vi "Test CAN read.vi"() -> ()   [LabVIEW 2023, in "PCAN API.lvlib"]
uses:
  PCAN API.lvlib
panel:
  out "MessageBuffer out 2":T1
  out "error out 3":errorcluster
  out "Array":errorcluster[](array[cluster])
  out "error out 2":errorcluster
  out "error out":errorcluster
  out "MessageBuffer out":T2(array[cluster])
  in  "stop":bool
  in  "error in":errorcluster
  in  "Channel":u16=81 format="%x"
  in  "IOPort":u32 format="%x"
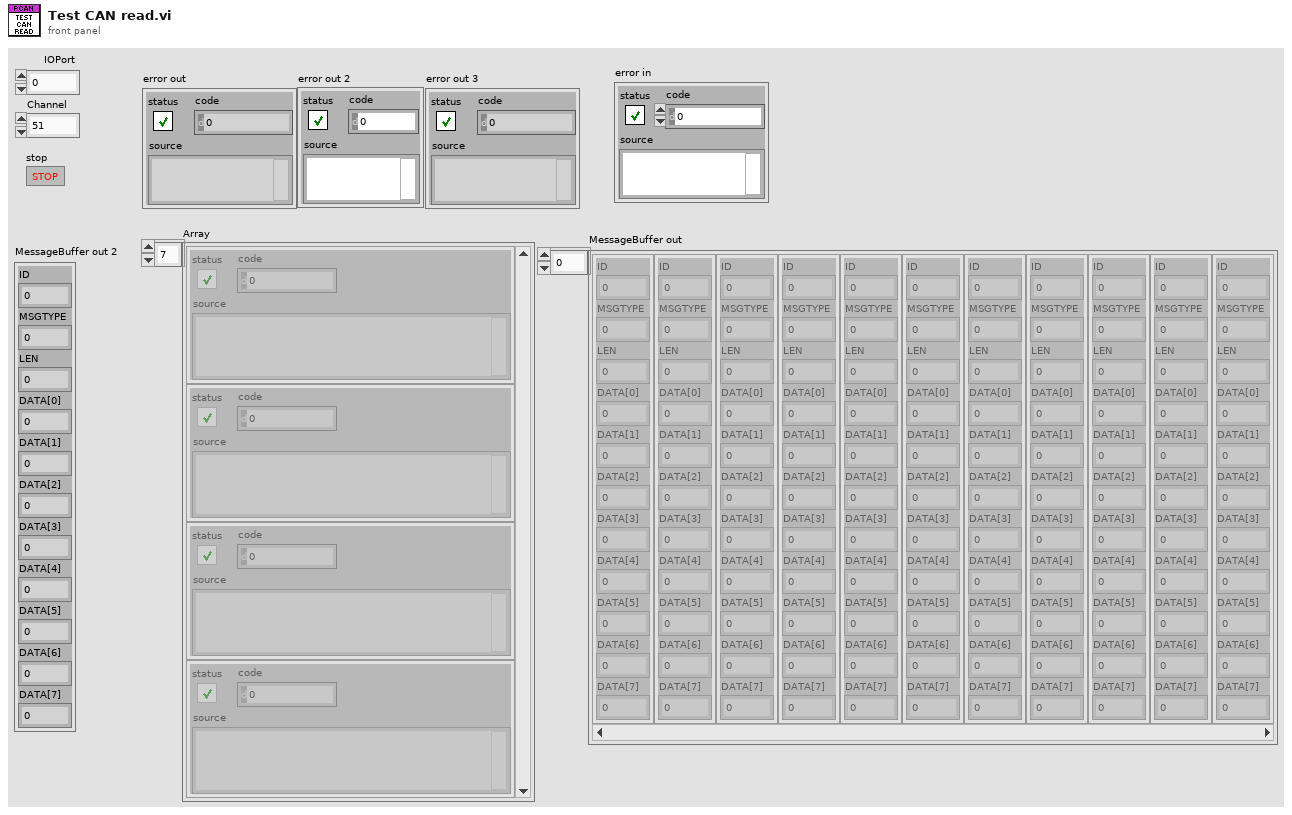
[diagram p1: front panel]
types:
  T1 = cluster{"ID":u32, "MSGTYPE":u8, "LEN":u8, "DATA[0]":u8, "DATA[1]":u8, "DATA[2]":u8, "DATA[3]":u8, "DATA[4]":u8, "DATA[5]":u8, "DATA[6]":u8, "DATA[7]":u8}
  T2 = cluster{"ID":u32, "MSGTYPE":u8, "LEN":u8, "DATA[0]":u8, "DATA[1]":u8, "DATA[2]":u8, "DATA[3]":u8, "DATA[4]":u8, "DATA[5]":u8, "DATA[6]":u8, "DATA[7]":u8}[]
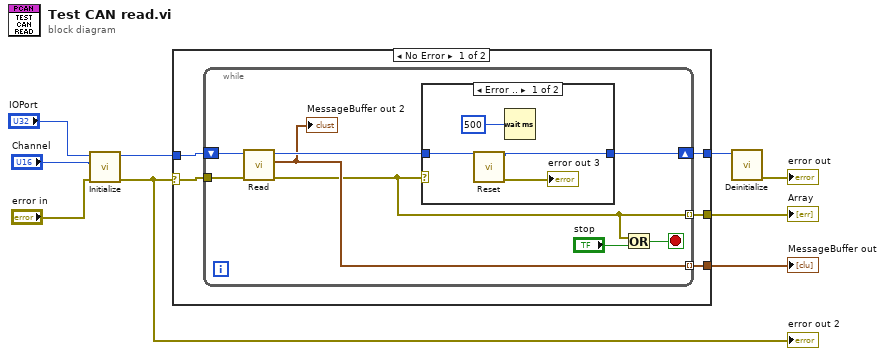
[diagram p0: block diagram]
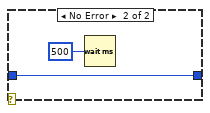
[diagram p2: hidden frame]
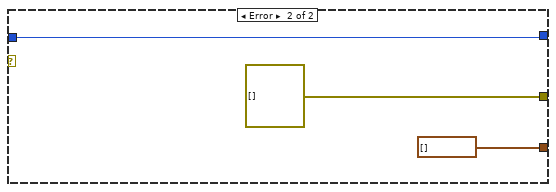
[diagram p3: hidden frame]
diagram:
  n1 = call "Initialize.vi"("error in"="error in", "Channel"="Channel", "IOPort"="IOPort") -> ("error out"=w7:errorcluster, "Channel"=w3:u16)  [unwired: 6 in, 1 out]
  "error out 2" <- w7
  n2 = case shown="No Error" w7 {
    selector: w7 -> [w12 _]
    tunnel: w3 -> [w14 w31]
    tunnel: [w13 w31] -> w9
    tunnel: [w11 errorcluster[] []] -> w2
    tunnel: [w10 T2 []] -> w1
    frame No Error {
      n3 = while {
        shift-right: [w19] -> w13
        shift-left: w14 -> [w22]
        tunnel: w12 -> [w21]
        tunnel: [w15] -> w11 mode=indexing
        tunnel: [w18] -> w10 mode=indexing
        stop <- w16 stop-if-true
        n4 = call "Read.vi"("error in"=w21, "Channel"=w22) -> ("error out"=w15:errorcluster, "MessageBuffer out"=w18:T1, "Channel out"=w20:u16)  [unwired: 6 in, 1 out]
        "MessageBuffer out 2" <- w18
        n5 = case shown="Error .." w15 {
          tunnel: w20 -> [w25 w28]
          tunnel: [w23 w28] -> w19
          frame Error {
            n6 = call "Reset.vi"("Channel"=w25) -> ("error out"=→"error out 3":errorcluster, "Channel out"=w23:u16)  [unwired: 9 in]
            n7 = Wait (ms)(milliseconds to wait=u32 500) -> ()  [unwired: 1 out]
          }
          frame No Error {
            n8 = Wait (ms)(milliseconds to wait=u32 500) -> ()  [unwired: 1 out]
          }
        }
        n9 = Or(x=w15, y="stop") -> (x .or. y?=w16:bool)
      }
    }
    frame Error {
    }
  }
  "Array" <- w2
  "MessageBuffer out" <- w1
  n10 = call "Deinitialize.vi"("Channel"=w9) -> ("error out"=→"error out":errorcluster)  [unwired: 10 in]
